vi "CalcDivSave.vi"() -> ()   [LabVIEW 2017]
panel:
  in  "Pixel size, um":dbl
  in  "Focus, mm":dbl
  in  "Rotate, deg":dbl=1.6 format="%#_13g"
  in  "Threshold, %":dbl=2.0 format="%#_13g"
  in  "path to PNG file":path=path "E:/New folder (3)/Laser(3dots)_FarField_after_Passive(WO_SAC).png"
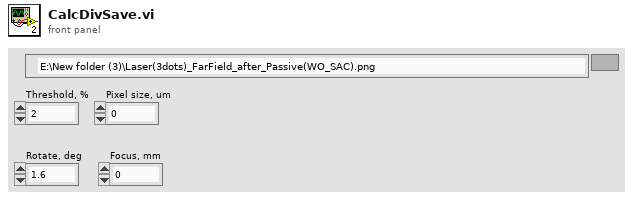
[diagram p1: front panel]
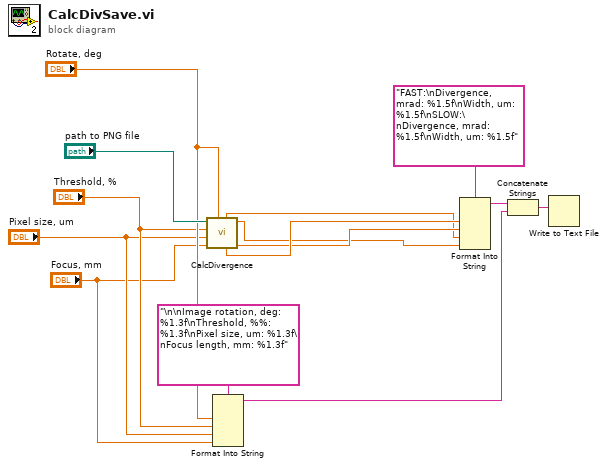
[diagram p0: block diagram]
diagram:
  n1 = call "CalcDivergence.vi"("Rotate, deg"="Rotate, deg", "Focus, mm"="Focus, mm", "Pixel size, um"="Pixel size, um", "Threshold, %"="Threshold, %", "path to PNG file"="path to PNG file") -> ("F Width, um"=w3:dbl, "S Width, um"=w1:dbl, "F Divergence, mrad"=w4:dbl, "S Divergence, mrad"=w2:dbl)  [unwired: 3 in]
  n2 = Format Into String(format string="\n\nImage rotation, deg: %1.3f\nThreshold, %%: %1.3f\nPixel size, um: %1.3f\nFocus length, mm: %1.3f", "Rotate, deg", "Threshold, %", "Pixel size, um", "Focus, mm") -> (resulting string=w6:string)  [unwired: 2 in, 1 out]
  n3 = Format Into String(format string="FAST:\nDivergence, mrad: %1.5f\nWidth, um: %1.5f\nSLOW:\nDivergence, mrad: %1.5f\nWidth, um: %1.5f", w4, w3, w2, w1) -> (resulting string=w7:string)  [unwired: 2 in, 1 out]
  n4 = Concatenate Strings(w7, w6) -> (w5:string)
  n5 = Write to Text File(text=w5) -> ()  [unwired: 3 in, 3 out]
